vi "VMC-2.vi"(11 "数组":u8[](array[numeric])) -> (1 "GLOADSST辅助数据有效字":T3, 2 "系统故障字1":T2, 3 "组合状态":T1, 4 "GPSBD辅助数据有效字":T4, 5 "组合模式受控状态":cluster{"自动":bool, " 强选":bool})   [LabVIEW 2012]
uses:
  index-i16.vi
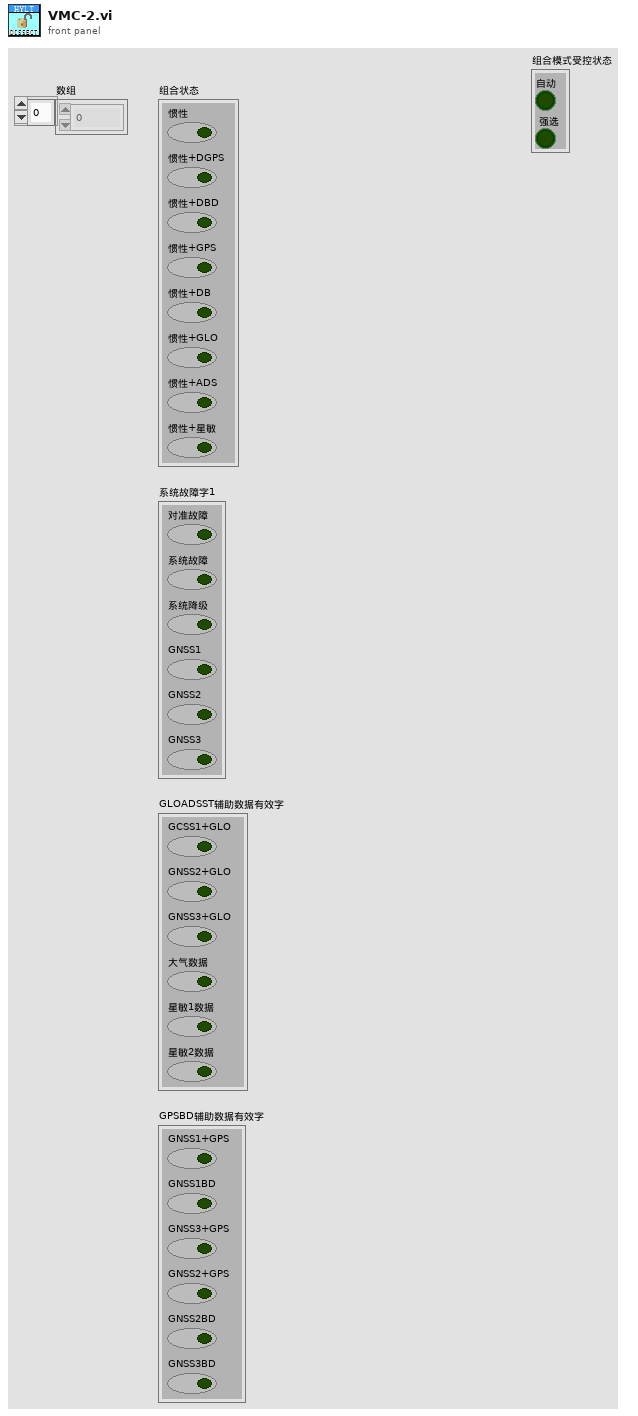
[diagram p1: front panel]
types:
  T1 = cluster{"惯性":bool, "惯性+DGPS":bool, "惯性+DBD":bool, "惯性+GPS":bool, "惯性+DB":bool, "惯性+GLO":bool, "惯性+ADS":bool, "惯性+星敏":bool}
  T2 = cluster{"对准故障":bool, "系统故障":bool, "系统降级":bool, "GNSS1":bool, "GNSS2":bool, "GNSS3":bool}
  T3 = cluster{"GCSS1+GLO":bool, "GNSS2+GLO":bool, "GNSS3+GLO":bool, "大气数据":bool, "星敏1数据":bool, "星敏2数据":bool}
  T4 = cluster{"GNSS1+GPS":bool, "GNSS1BD":bool, "GNSS3+GPS":bool, "GNSS2+GPS":bool, "GNSS2BD":bool, "GNSS3BD":bool}
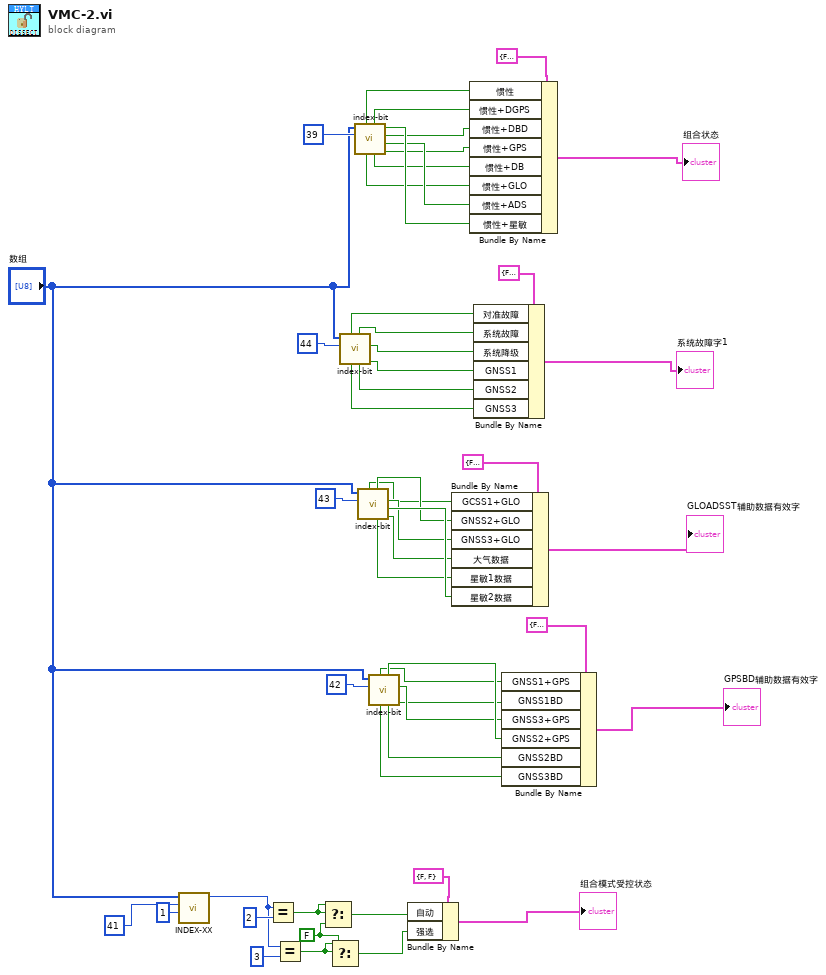
[diagram p0: block diagram]
diagram:
  w1 = FALSE ("f")
  n1 = call-poly "INDEX-XX.vi"("长度"=1, "索引"=41, "数组"="数组") -> ("数值输出"=w2:i16)  [unwired: 8 in]
  n2 = Equal?(x=w2, y=u8 2) -> (x = y?=w10:bool)
  n3 = Equal?(x=w2, y=u8 3) -> (x = y?=w9:bool)
  n4 = Select(t=w10, s=w10, f=w1) -> (s? t:f=w11:bool)
  n5 = Select(t=w9, s=w9, f=w1) -> (s? t:f=w7:bool)
  n6 = call "index-bit.vi"("index"=44 ("索引"), "array"="数组") -> ("bit3"=w28:bool, "bit2"=w27:bool, "bit4"=w29:bool, "bit1"=w26:bool, "bit5"=w30:bool, "bit0"=w25:bool)  [unwired: 2 in, 2 out]
  n7 = call "index-bit.vi"("index"=39 ("索引"), "array"="数组") -> ("bit3"=w19:bool, "bit6"=w22:bool, "bit2"=w18:bool, "bit7"=w23:bool, "bit4"=w20:bool, "bit1"=w17:bool, "bit5"=w21:bool, "bit0"=w16:bool)  [unwired: 2 in]
  n8 = call "index-bit.vi"("index"=43 ("索引"), "array"="数组") -> ("bit3"=w40:bool, "bit6"=w42:bool, "bit2"=w39:bool, "bit4"=w41:bool, "bit1"=w38:bool, "bit0"=w37:bool)  [unwired: 2 in, 2 out]
  n9 = call "index-bit.vi"("index"=42 ("索引"), "array"="数组") -> ("bit3"=w47:bool, "bit2"=w48:bool, "bit4"=w50:bool, "bit1"=w49:bool, "bit5"=w51:bool, "bit0"=w46:bool)  [unwired: 2 in, 2 out]
  n10 = Bundle By Name(cluster=cluster{"自动":bool, " 强选":bool} {"自动"=FALSE, " 强选"=FALSE} ("组合模式受控状态"), "自动"=w11, "强选"=w7) -> (→"组合模式受控状态":cluster{"自动":bool, " 强选":bool})
  n11 = Bundle By Name(cluster=T3 {"GCSS1+GLO"=FALSE, "GNSS2+GLO"=FALSE, "GNSS3+GLO"=FALSE, "大气数据"=FALSE, "星敏1数据"=FALSE, "星敏2数据"=FALSE} ("GLOADSST辅助数据有效字"), "GCSS1+GLO"=w37, "GNSS2+GLO"=w38, "GNSS3+GLO"=w39, "大气数据"=w40, "星敏1数据"=w41, "星敏2数据"=w42) -> (→"GLOADSST辅助数据有效字":T3)
  n12 = Bundle By Name(cluster=T1 {"惯性"=FALSE, "惯性+DGPS"=FALSE, "惯性+DBD"=FALSE, "惯性+GPS"=FALSE, "惯性+DB"=FALSE, "惯性+GLO"=FALSE, "惯性+ADS"=FALSE, "惯性+星敏"=FALSE} ("组合状态"), "惯性"=w16, "惯性+DGPS"=w17, "惯性+DBD"=w18, "惯性+GPS"=w19, "惯性+DB"=w20, "惯性+GLO"=w21, "惯性+ADS"=w22, "惯性+星敏"=w23) -> (→"组合状态":T1)
  n13 = Bundle By Name(cluster=T2 {"对准故障"=FALSE, "系统故障"=FALSE, "系统降级"=FALSE, "GNSS1"=FALSE, "GNSS2"=FALSE, "GNSS3"=FALSE} ("系统故障"), "对准故障"=w25, "系统故障"=w26, "系统降级"=w27, "GNSS1"=w28, "GNSS2"=w29, "GNSS3"=w30) -> (→"系统故障字1":T2)
  n14 = Bundle By Name(cluster=T4 {"GNSS1+GPS"=FALSE, "GNSS1BD"=FALSE, "GNSS3+GPS"=FALSE, "GNSS2+GPS"=FALSE, "GNSS2BD"=FALSE, "GNSS3BD"=FALSE} ("GPSBD辅助数据有效字"), "GNSS1+GPS"=w46, "GNSS1BD"=w47, "GNSS3+GPS"=w48, "GNSS2+GPS"=w49, "GNSS2BD"=w50, "GNSS3BD"=w51) -> (→"GPSBD辅助数据有效字":T4)
